vi "soliton-trigger-final-rf.vi"() -> ()   [LabVIEW 2015]
doc: "This example demonstrates how to generate a single pulse using a counter output. \n\nThe single pulse may be triggered once or repeatedly from an external source."
uses:
  <vilib>/Utility/error.llb/DialogType.ctl
  <vilib>/DAQmx/create/channels.llb/DAQmx Create Channel (CO-Pulse Generation-Time).vi
  <resource>/objmgr/daqmx.rc
panel:
  in  "soliton higher bound":dbl=0.05
  in  "soliton lower bound":dbl=-0.05
  in  "ms to start diagnose":u32=100
  out "Comb Power monitor":dbl=-1.3606006170113327
  in  "Pulse Duration 2":dbl=0.001 format="%.6f"
  in  "Output Terminal 2":tag="/Dev1/PFI0"
  in  "Counter 2":tag="Dev1/ctr0"
  out "Number of diagnose":i32=583
  out "Trigger?":bool=TRUE
  in  "stop":bool
  in  "Stop":bool
  # "Channel Settings"
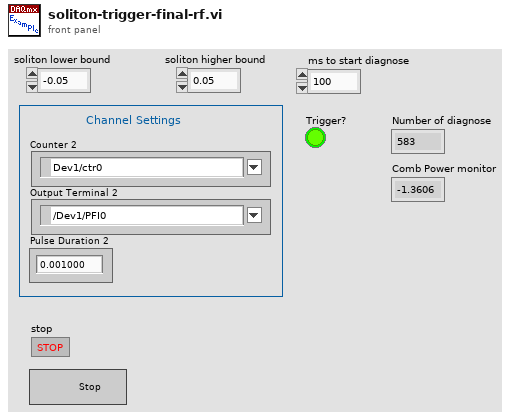
[diagram p1: front panel]
types:
  T1 = typedef "DialogType.ctl" = u16
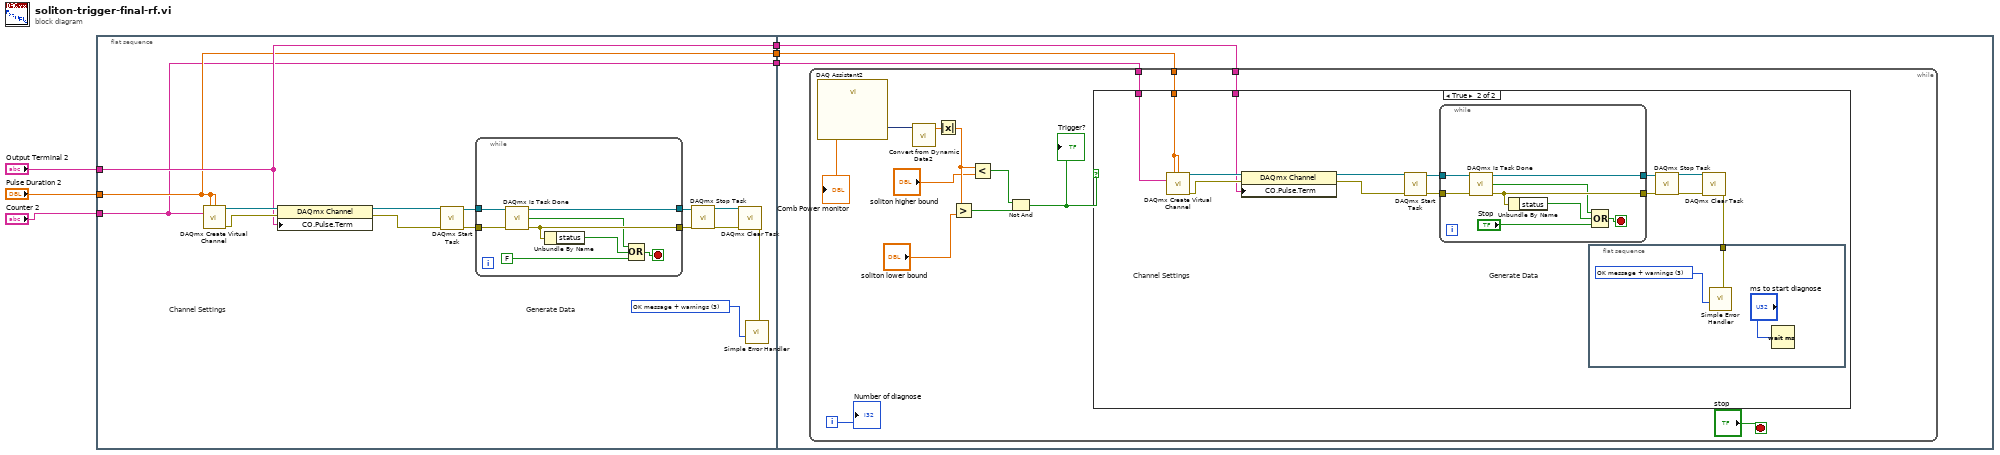
[diagram p0: block diagram]
diagram:
  n1 = flat-sequence {
    tunnel: "Output Terminal 2" -> [w9]
    tunnel: "Counter 2" -> [w7]
    tunnel: "Pulse Duration 2" -> [w8]
    tunnel: [w9] -> w3
    tunnel: [w8] -> w2
    tunnel: [w7] -> w1
    tunnel: w3 -> [w32]
    tunnel: w2 -> [w31]
    tunnel: w1 -> [w30]
    frame #0 {
      w12 = T1 3 items=["no dialog", "OK message", "continue or stop message", "OK message + warnings", "continue/stop + warnings"] ("type of dialog (OK msg:1)")
      # "Generate Data"
      # "Channel Settings"
      n2 = call-poly <vilib>:"DAQmx Create Virtual Channel.vi"("high time"=w8, "low time"=w8, "counter"=w7) -> ("task out"=w18:refnum<k21>, "error out"=w17:errorcluster)  [unwired: 11 in]
      n3 = property class="DAQmx Channel"(reference=w18, error in=w17, "CO.Pulse.Term"=w9) -> (reference out=w10:refnum<k21>, error out=w11:errorcluster)
      n4 = call <vilib>:"DAQmx Start Task.vi"("task/channels in"=w10, "error in"=w11) -> ("task out"=w21:refnum<k21>, "error out"=w20:errorcluster)  [unwired: 12 in]
      n5 = while {
        tunnel: w21 -> [w29]
        tunnel: w20 -> [w28]
        tunnel: [w25] -> w15
        tunnel: [w26] -> w16
        stop <- w27 stop-if-true
        n6 = call <vilib>:"DAQmx Is Task Done.vi"("task/channels in"=w29, "error in"=w28) -> ("task out"=w26:refnum<k21>, "task done?"=w22:bool, "error out"=w25:errorcluster)  [unwired: 11 in]
        n7 = Unbundle By Name(w25) -> ("status"=w24:bool)
        n8 = Compound Arithmetic op=OR(w22, w24, FALSE ("Stop 2")) -> (w27:bool)
      }
      n9 = call <vilib>:"DAQmx Stop Task.vi"("task/channels in"=w16, "error in"=w15) -> ("task out"=w14:refnum<k21>, "error out"=w13:errorcluster)  [unwired: 12 in]
      n10 = call <vilib>:"DAQmx Clear Task.vi"("task in"=w14, "error in"=w13) -> ("error out"=w19:errorcluster)  [unwired: 13 in]
      n11 = call <vilib>:"Simple Error Handler.vi"("type of dialog (OK msg:1)"=w12, "error in (no error)"=w19) -> ()  [unwired: 3 in, 5 out]
    }
    frame #1 {
      n12 = while {
        tunnel: w32 -> [w43]
        tunnel: w31 -> [w42]
        tunnel: w30 -> [w41]
        i -> [w40]
        stop <- "stop" stop-if-true
        n13 = call "DAQ Assistant2"() -> ("data"=w44:dynamicdata)  [unwired: 17 in, 2 out]
        n14 = call "Convert from Dynamic Data2"("Dynamic Data Type"=w44) -> ("Scalar"=w39:dbl)  [unwired: 3 in]
        "Comb Power monitor" <- w39
        n15 = Absolute Value(x=w39) -> (abs(x)=w37:dbl)
        n16 = Greater?(x=w37, y="soliton lower bound") -> (0:w34:bool)
        n17 = Less?(x=w37, y="soliton higher bound") -> (x < y?=w35:bool)
        n18 = Not And(1:w34, 2:w35) -> (0:w33:bool)
        "Trigger?" <- w33
        n19 = case shown="True" w33 {
          tunnel: w43 -> [_ w48]
          tunnel: w42 -> [_ w47]
          tunnel: w41 -> [_ w46]
          frame False {
          }
          frame True {
            # "Generate Data"
            # "Channel Settings"
            n20 = call-poly <vilib>:"DAQmx Create Virtual Channel.vi"("high time"=w47, "low time"=w47, "counter"=w46) -> ("task out"=w56:refnum<k21>, "error out"=w55:errorcluster)  [unwired: 11 in]
            n21 = property class="DAQmx Channel"(reference=w56, error in=w55, "CO.Pulse.Term"=w48) -> (reference out=w49:refnum<k21>, error out=w50:errorcluster)
            n22 = call <vilib>:"DAQmx Start Task.vi"("task/channels in"=w49, "error in"=w50) -> ("task out"=w59:refnum<k21>, "error out"=w58:errorcluster)  [unwired: 12 in]
            n23 = while {
              tunnel: w59 -> [w70]
              tunnel: w58 -> [w69]
              tunnel: [w66] -> w53
              tunnel: [w67] -> w54
              stop <- w68 stop-if-true
              n24 = call <vilib>:"DAQmx Is Task Done.vi"("task/channels in"=w70, "error in"=w69) -> ("task out"=w67:refnum<k21>, "task done?"=w63:bool, "error out"=w66:errorcluster)  [unwired: 11 in]
              n25 = Unbundle By Name(w66) -> ("status"=w65:bool)
              n26 = Compound Arithmetic op=OR(w63, w65, "Stop") -> (w68:bool)
            }
            n27 = flat-sequence {
              tunnel: w57 -> [w62]
              frame #0 {
                w61 = T1 3 items=["no dialog", "OK message", "continue or stop message", "OK message + warnings", "continue/stop + warnings"] ("type of dialog (OK msg:1)")
                n28 = call <vilib>:"Simple Error Handler.vi"("type of dialog (OK msg:1)"=w61, "error in (no error)"=w62) -> ()  [unwired: 3 in, 5 out]
                n29 = Wait (ms)(milliseconds to wait="ms to start diagnose") -> ()  [unwired: 1 out]
              }
            }
            n30 = call <vilib>:"DAQmx Stop Task.vi"("task/channels in"=w54, "error in"=w53) -> ("task out"=w52:refnum<k21>, "error out"=w51:errorcluster)  [unwired: 12 in]
            n31 = call <vilib>:"DAQmx Clear Task.vi"("task in"=w52, "error in"=w51) -> ("error out"=w57:errorcluster)  [unwired: 13 in]
          }
        }
        "Number of diagnose" <- w40
      }
    }
  }
